vi "Add Field to Cluster.vi"(9 "Field Name":string, 10 "Cluster":refnum<vi>, 11 "Abstract Param Writer in":refnum<class "Abstract Param Writer.lvclass">) -> (2 "Cluster Dup":refnum<vi>, 3 "Abstract Param Writer out":refnum<class "Abstract Param Writer.lvclass">)   [LabVIEW 2013, in "Abstract Param Writer.lvclass"]
uses:
  Abstract Param Writer.lvclass
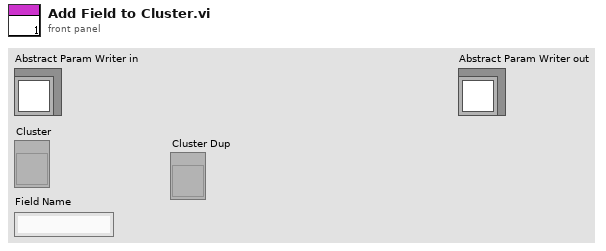
[diagram p1: front panel]
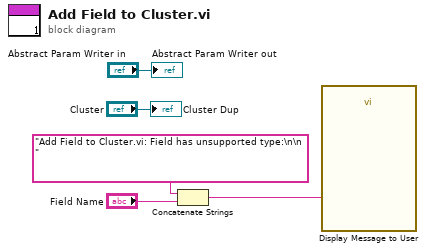
[diagram p0: block diagram]
diagram:
  n1 = Concatenate Strings("Add Field to Cluster.vi: Field has unsupported type:\n\n    ", "Field Name") -> (w2:string)
  n2 = call "Display Message to User"("Message"=w2) -> ()  [unwired: 9 in, 2 out]
  "Abstract Param Writer out" <- "Abstract Param Writer in"
  "Cluster Dup" <- "Cluster"
